vi "DuALEX_RG.vi"() -> ()   [LabVIEW 2011]
uses:
  <vilib>/DAQmx/write.llb/DAQmx Write (Analog Wfm 1Chan NSamp).vi
  <vilib>/DAQmx/create/channels.llb/DAQmx Create Channel (AO-Voltage-Basic).vi
  <vilib>/DAQmx/configure/timing.llb/DAQmx Timing (Sample Clock).vi
  <vilib>/DAQmx/create/channels.llb/DAQmx Create Channel (CO-Pulse Generation-Frequency).vi
  <vilib>/DAQmx/configure/events/hardwareSignals.llb/DAQmx Export Signal (Most Signals).vi
  <vilib>/DAQmx/configure/trigger.llb/DAQmx Start Trigger (Digital Edge).vi
  <vilib>/DAQmx/configure/timing.llb/DAQmx Timing (Implicit).vi
  <vilib>/DAQmx/miscellaneous.llb/DAQmx Fill In Error Info.vi
  <vilib>/measure/NI_MABase.lvlib
panel:
  in  "Analog Amplitude":dbl=1.0 format="%0.2p"
  in  "Repetition Frequency":dbl=1.0 format="%.6f"
  in  "Stop Button":bool
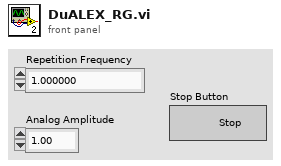
[diagram p1: front panel]
types:
  T1 = enum16{"Sine Wave", "Triangle Wave", "Square Wave", "Sawtooth Wave"}
  T2 = cluster{"Ao0 Sample Clock Rate":dbl, "Ao0 Sample Clock Rate":dbl}
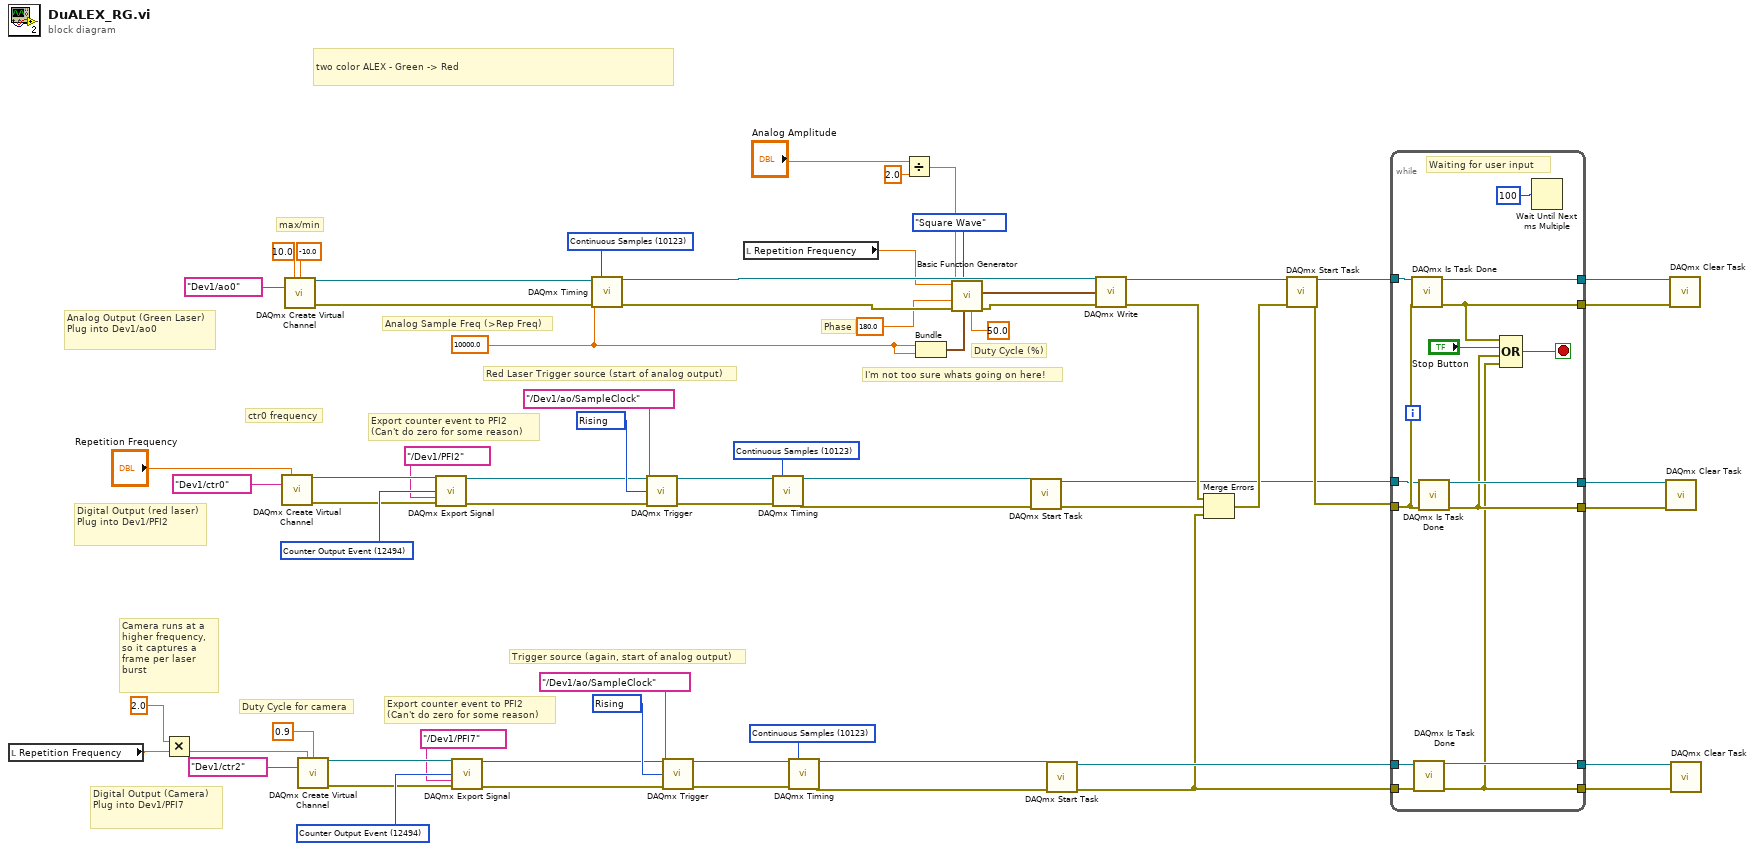
[diagram p0: block diagram]
diagram:
  w18 = 10280 items=["Rising"=10280, "Falling"=10171] ("edge")
  w21 = 10123 items=["Finite Samples"=10178, "Continuous Samples"=10123, "Hardware Timed Single Point"=12522] ("sample mode")
  w23 = 12494 items=["AI Convert Clock"=12484, "10MHz Reference Clock"=12536, "20MHz Timebase Clock"=12486, "Sample Clock"=12487, "Advance Trigger"=12488, "Reference Trigger"=12490, "Start Trigger"=12491, "Advance Complete Event"=12492, "AI Hold Complete Event"=12493, "Counter Output Event"=12494, "Change Detection Event"=12511, "Watchdog Timer Expired Event"=12512] ("signal")
  w32 = 10123 items=["Finite Samples"=10178, "Continuous Samples"=10123, "Hardware Timed Single Point"=12522] ("sample mode")
  w54 = 10280 items=["Rising"=10280, "Falling"=10171] ("edge")
  w59 = 10123 items=["Finite Samples"=10178, "Continuous Samples"=10123, "Hardware Timed Single Point"=12522] ("sample mode")
  w61 = 12494 items=["AI Convert Clock"=12484, "10MHz Reference Clock"=12536, "20MHz Timebase Clock"=12486, "Sample Clock"=12487, "Advance Trigger"=12488, "Reference Trigger"=12490, "Start Trigger"=12491, "Advance Complete Event"=12492, "AI Hold Complete Event"=12493, "Counter Output Event"=12494, "Change Detection Event"=12511, "Watchdog Timer Expired Event"=12512] ("signal")
  w1 = 10000.0 ("Ao0 Sample Clock Rate")
  # "two color ALEX - Green -> Red"
  # "Duty Cycle for camera"
  # "Camera runs at a higher frequency, so it captures a frame per laser burst"
  # "Digital Output (Camera) Plug into Dev1/PFI7"
  # "Trigger source (again, start of analog output)"
  # "Export counter event to PFI2\n(Can't do zero for some reason)"
  # "Digital Output (red laser) Plug into Dev1/PFI2"
  # "Analog Output (Green Laser) Plug into Dev1/ao0"
  # "Duty Cycle (%)"
  # "Phase"
  # "Analog Sample Freq (>Rep Freq)"
  # "I'm not too sure whats going on here!"
  # "Red Laser Trigger source (start of analog output)"
  # "Export counter event to PFI2\n(Can't do zero for some reason)"
  # "ctr0 frequency"
  # "max/min"
  n1 = local read "Repetition Frequency"() -> (w10:dbl)
  n2 = Multiply(x=2.0 ("Repetition Frequency"), y=w10) -> (x*y=w9:dbl)
  n3 = call-poly <vilib>:"DAQmx Create Virtual Channel.vi"("frequency"="Repetition Frequency", "counter"=tag "Dev1/ctr0") -> ("task out"=w62:refnum<k21>, "error out"=w60:errorcluster)  [unwired: 12 in]
  n4 = call-poly <vilib>:"DAQmx Create Virtual Channel.vi"("maximum value"=10.0, "minimum value"=-10.0, "physical channels"=tag "Dev1/ao0") -> ("task out"=w66:refnum<k21>, "error out"=w65:errorcluster)  [unwired: 11 in]
  n5 = call-poly <vilib>:"DAQmx Create Virtual Channel.vi"("frequency"=w9, "duty cycle"=0.9, "counter"=tag "Dev1/ctr2") -> ("task out"=w24:refnum<k21>, "error out"=w22:errorcluster)  [unwired: 11 in]
  n6 = call-poly <vilib>:"DAQmx Export Signal.vi"("task/channels in"=w62, "signal"=w61, "output terminal"=tag "/Dev1/PFI2", "error in"=w60) -> ("task out"=w53:refnum<k21>, "error out"=w50:errorcluster)  [unwired: 10 in]
  n7 = call-poly <vilib>:"DAQmx Export Signal.vi"("task/channels in"=w24, "signal"=w23, "output terminal"=tag "/Dev1/PFI7", "error in"=w22) -> ("task out"=w17:refnum<k21>, "error out"=w14:errorcluster)  [unwired: 10 in]
  n8 = call-poly <vilib>:"DAQmx Timing.vi"("task/channels in"=w66, "sample mode"=w32, "rate"=w1, "error in"=w65) -> ("task out"=w58:refnum<k21>, "error out"=w57:errorcluster)  [unwired: 10 in]
  n9 = call-poly <vilib>:"DAQmx Trigger.vi"("task/channels in"=w53, "source"=tag "/Dev1/ao/SampleClock", "edge"=w54, "error in"=w50) -> ("task out"=w52:refnum<k21>, "error out"=w51:errorcluster)  [unwired: 10 in]
  n10 = call-poly <vilib>:"DAQmx Trigger.vi"("task/channels in"=w17, "source"=tag "/Dev1/ao/SampleClock", "edge"=w18, "error in"=w14) -> ("task out"=w16:refnum<k21>, "error out"=w15:errorcluster)  [unwired: 10 in]
  n11 = local read "Repetition Frequency"() -> (w29:dbl)
  n12 = call-poly <vilib>:"DAQmx Timing.vi"("task/channels in"=w52, "sample mode"=w59, "error in"=w51) -> ("task out"=w46:refnum<k21>, "error out"=w45:errorcluster)  [unwired: 11 in]
  n13 = call-poly <vilib>:"DAQmx Timing.vi"("task/channels in"=w16, "sample mode"=w21, "error in"=w15) -> ("task out"=w13:refnum<k21>, "error out"=w12:errorcluster)  [unwired: 11 in]
  n14 = Divide(x="Analog Amplitude", y=2.0) -> (x/y=w26:dbl)
  n15 = Bundle("Ao0 Sample Clock Rate"=w1, "Ao0 Sample Clock Rate"=w1) -> (w2:T2)  [unwired: 1 in]
  n16 = call <vilib>:"Basic Function Generator.vi"("offset"=w26, "square wave duty cycle (%)"=50.0, "sampling info"=w2, "signal type"=T1."Square Wave", "error in (no error)"=w57, "phase"=180.0, "amplitude"=w26, "frequency"=w29) -> ("error out"=w48:errorcluster, "signal out"=w49:waveform(dbl))  [unwired: 1 in, 1 out]
  n17 = call <vilib>:"DAQmx Start Task.vi"("task/channels in"=w46, "error in"=w45) -> ("task out"=w33:refnum<k21>, "error out"=w44:errorcluster)  [unwired: 12 in]
  n18 = call <vilib>:"DAQmx Start Task.vi"("task/channels in"=w13, "error in"=w12) -> ("task out"=w6:refnum<k21>, "error out"=w5:errorcluster)  [unwired: 12 in]
  n19 = call-poly <vilib>:"DAQmx Write.vi"("task/channels in"=w58, "data"=w49, "error in"=w48) -> ("task out"=w41:refnum<k21>, "error out"=w43:errorcluster)  [unwired: 10 in, 1 out]
  n20 = Merge Errors(w43, w44, w5) -> (w42:errorcluster)
  n21 = call <vilib>:"DAQmx Start Task.vi"("task/channels in"=w41, "error in"=w42) -> ("task out"=w39:refnum<k21>, "error out"=w38:errorcluster)  [unwired: 12 in]
  n22 = while {
    tunnel: [w81] -> w34
    tunnel: [w72] -> w37
    tunnel: [w78] -> w35
    tunnel: [w70] -> w36
    tunnel: w39 -> [w77]
    tunnel: w38 -> [w76]
    tunnel: w33 -> [w75]
    tunnel: w6 -> [w74]
    tunnel: w5 -> [w73]
    tunnel: [w69] -> w4
    tunnel: [w68] -> w3
    stop <- w79 stop-if-true
    # "Waiting for user input"
    n23 = call <vilib>:"DAQmx Is Task Done.vi"("task/channels in"=w77, "error in"=w76) -> ("task out"=w81:refnum<k21>, "error out"=w72:errorcluster)  [unwired: 11 in, 1 out]
    n24 = call <vilib>:"DAQmx Is Task Done.vi"("task/channels in"=w74, "error in"=w73) -> ("task out"=w69:refnum<k21>, "error out"=w68:errorcluster)  [unwired: 11 in, 1 out]
    n25 = call <vilib>:"DAQmx Is Task Done.vi"("task/channels in"=w75, "error in"=w76) -> ("task out"=w78:refnum<k21>, "error out"=w70:errorcluster)  [unwired: 11 in, 1 out]
    n26 = Compound Arithmetic op=OR(w72, "Stop Button", w70, w68) -> (w79:bool)
    n27 = Wait Until Next ms Multiple(millisecond multiple=u32 100) -> ()  [unwired: 1 out]
  }
  n28 = call <vilib>:"DAQmx Clear Task.vi"("task in"=w35, "error in"=w36) -> ()  [unwired: 13 in, 1 out]
  n29 = call <vilib>:"DAQmx Clear Task.vi"("task in"=w34, "error in"=w37) -> ()  [unwired: 13 in, 1 out]
  n30 = call <vilib>:"DAQmx Clear Task.vi"("task in"=w4, "error in"=w3) -> ()  [unwired: 13 in, 1 out]
